vi "Set VI Probes.vi"(8 "error in":errorcluster, 10 "Probes":i32[](array[numeric]), 11 "VI Reference in":refnum<vi>) -> (0 "error out":errorcluster, 2 "VI Modified":bool, 3 "VI Reference out":refnum<vi>)   [LabVIEW 2020]
doc: "This VI sets probes in wires with the provided <b>UIDs</b> of the active VI."
uses:
  <vilib>/Utility/traverseref.llb/TRef TravTarget.ctl
  Type Definitions/Class Name--enum.ctl
  <vilib>/Utility/traverseref.llb/VI Scripting - Traverse.lvlib
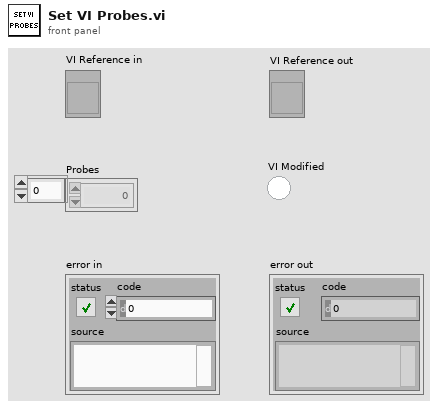
[diagram p1: front panel]
types:
  T1 = typedef "Class Name--enum.ctl" = enum16{"Node", "Wire"}
  T2 = typedef "TRef TravTarget.ctl" = enum16{"FP", "BD", "Other"}
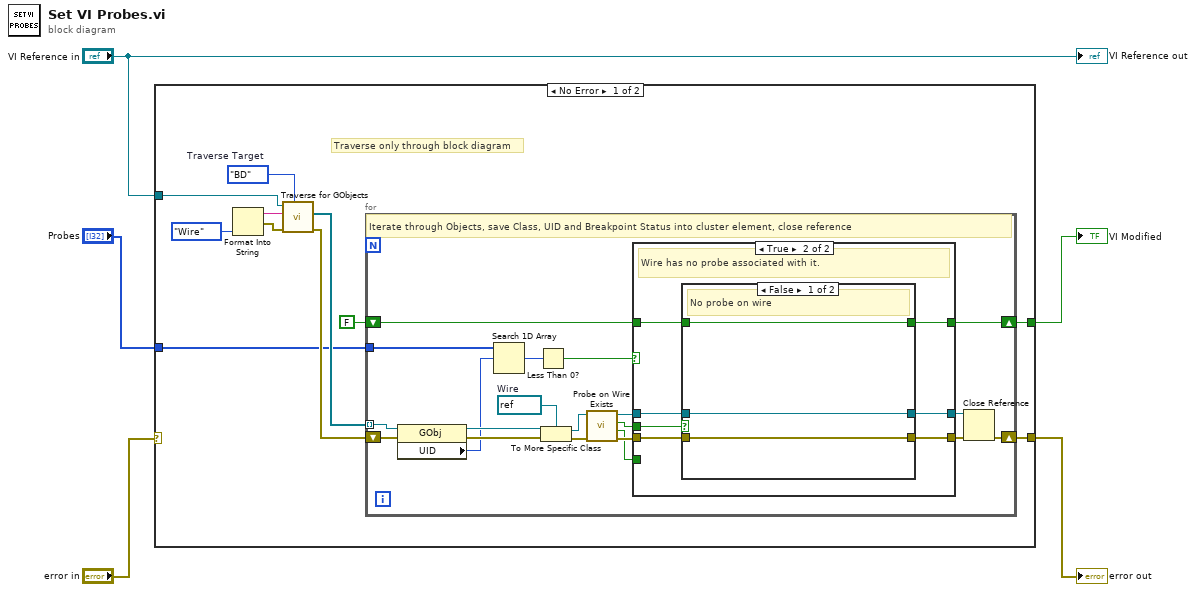
[diagram p0: block diagram]
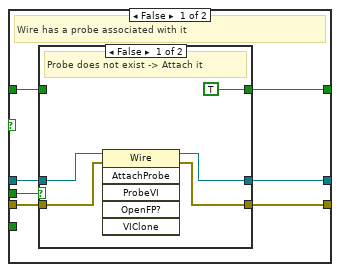
[diagram p2: hidden frame]
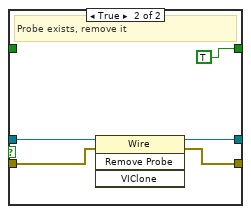
[diagram p4: hidden frame]
diagram:
  n1 = case shown="No Error" "error in" {
    selector: "error in" -> [_ w67]
    tunnel: "VI Reference in" -> [w13 _]
    tunnel: [w14 w67] -> w4
    tunnel: "Probes" -> [w8 _]
    tunnel: [w6 _] -> w2
    frame No Error {
      w12 = TRef_TravTarget."BD"  # Traverse Target
      # "Traverse only through block diagram"
      n2 = Format Into String(Class_Name--enum."Wire" ("Class Name")) -> (resulting string=w10:string, error out=w15:errorcluster)  [unwired: 3 in]
      n3 = call <vilib>:"Traverse for GObjects.vi"("Traverse Target"=w12, "error in (no error)"=w15, "Class Name"=w10, "VI Refnum"=w13) -> ("error out"=w16:errorcluster, "References"=w11:refnum<vi>[])  [unwired: 4 in, 2 out]
      n4 = for {
        tunnel: w11 -> [w30] mode=indexing
        shift-right: [w35] -> w14
        shift-left: w16 -> [w36]
        tunnel: w8 -> [w28]
        shift-right: [w21] -> w6
        shift-left: FALSE -> [w22]
        w23 = refnum<vi> refnum  # Wire
        # "Iterate through Objects, save Class, UID and Breakpoint Status into cluster element, close reference"
        n5 = property class="GObj"(reference=w30, error in=w36) -> (reference out=w29:refnum<vi>, error out=w33:errorcluster, "UID"=w27:i32)
        n6 = Search 1D Array(1D array=w28, element=w27) -> (index of element=w26:i32)  [unwired: 1 in]
        n7 = Less Than 0?(x=w26) -> (x < 0?=w25:bool)
        n8 = To More Specific Class(target class=w23, reference=w29, error in=w33) -> (specific class reference=w20:refnum<vi>, error out=w32:errorcluster)
        n9 = call "Probe on Wire Exists.vi"("error in"=w32, "Wire in"=w20) -> ("error out"=w31:errorcluster, "Dummy Output"=w17:bool, "Probe Exists"=w18:bool, "Wire out"=w19:refnum<vi>)  [unwired: 6 in]
        n10 = case shown="True" w25 {
          tunnel: w31 -> [w42 w58]
          tunnel: [w43 w57] -> w34
          tunnel: [w41 w55] -> w24
          tunnel: w19 -> [w38 w56]
          tunnel: w22 -> [w40 w52]
          tunnel: [w39 w53] -> w21
          tunnel: w18 -> [w37 w54]
          tunnel: w17 -> [_ _]
          frame False {
            # "Wire has a probe associated with it"
            n11 = case shown="False" w37 {
              tunnel: [w46 w50] -> w41
              tunnel: [w48 w51] -> w43
              tunnel: w42 -> [w47 w51]
              tunnel: w38 -> [w45 w50]
              tunnel: w40 -> [_ w49]
              tunnel: [TRUE w49] -> w39
              frame False {
                # "Probe does not exist -> Attach it"
                n12 = invoke class="Wire" method="AttachProbe"(reference=w45, error in=w47) -> (reference out=w46:refnum<vi>, error out=w48:errorcluster)  [unwired: 4 in, 4 out]
              }
              frame True {
                # "Probe already exists"
              }
            }
          }
          frame True {
            # "Wire has no probe associated with it."
            n13 = case shown="False" w54 {
              tunnel: w56 -> [w59 w64]
              tunnel: [w59 w63] -> w55
              tunnel: w58 -> [w61 w66]
              tunnel: [w61 w65] -> w57
              tunnel: [w60 TRUE] -> w53
              tunnel: w52 -> [w60 _]
              frame False {
                # "No probe on wire"
              }
              frame True {
                # "Probe exists, remove it"
                n14 = invoke class="Wire" method="Remove Probe"(reference=w64, error in=w66) -> (reference out=w63:refnum<vi>, error out=w65:errorcluster)  [unwired: 2 in, 2 out]
              }
            }
          }
        }
        n15 = Close Reference(reference=w24, error in (no error)=w34) -> (error out=w35:errorcluster)
      }
    }
    frame Error {
      # "Pass error without further action"
    }
  }
  "error out" <- w4
  "VI Modified" <- w2
  "VI Reference out" <- "VI Reference in"
